vi "bd_bounds.vi"(8 "error in (no error)":errorcluster, 11 "VI Refnum":refnum<vi>) -> (0 "error out":errorcluster, 3 "VI Refnum Out":refnum<vi>)   [LabVIEW 2018]
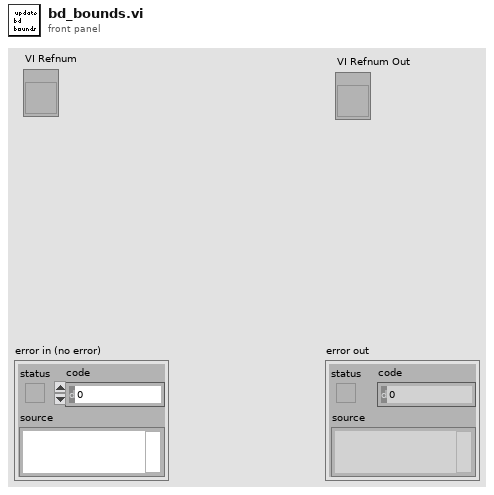
[diagram p1: front panel]
types:
  T1 = typedef "LVRectTypeDef.ctl" = cluster{"Left":i16, "Top":i16, "Right":i16, "Bottom":i16}
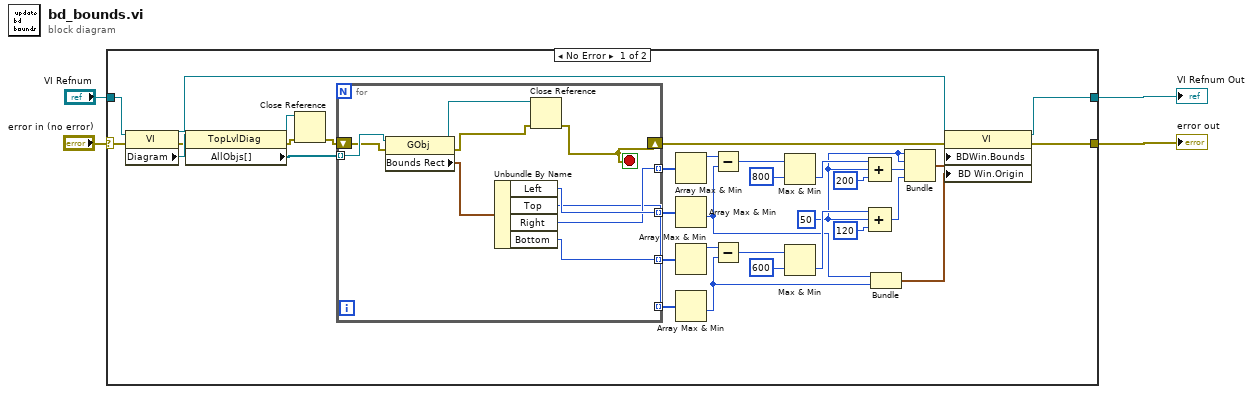
[diagram p0: block diagram]
diagram:
  n1 = case shown="No Error" "error in (no error)" {
    selector: "error in (no error)" -> [w21 w48]
    tunnel: "VI Refnum" -> [w37 w49]
    tunnel: [w12 w49] -> w3
    tunnel: [w5 w48] -> w1
    frame No Error {
      w26 = 50
      n2 = property class="VI"(reference=w37, error in=w21) -> (reference out=w29:refnum<vi>, error out=w20:errorcluster, "Diagram"=w36:refnum<vi>)
      n3 = property class="TopLvlDiag"(reference=w36, error in=w20) -> (reference out=w9:refnum<vi>, error out=w11:errorcluster, "AllObjs[]"=w35:refnum<vi>[])
      n4 = Close Reference(reference=w9, error in (no error)=w11) -> (error out=w10:errorcluster)
      n5 = for {
        tunnel: w35 -> [w47] mode=indexing
        tunnel: [w46] -> w34 mode=indexing
        tunnel: [w42] -> w33 mode=indexing
        shift-right: [w38] -> w22
        shift-left: w10 -> [w43]
        tunnel: [w45] -> w17 mode=indexing
        tunnel: [w44] -> w15 mode=indexing
        stop <- w38 stop-if-true
        n6 = property class="GObj"(reference=w47, error in=w43) -> (reference out=w39:refnum<vi>, error out=w40:errorcluster, "Bounds Rect"=w41:T1)
        n7 = Unbundle By Name(w41) -> ("Left"=w46:i16, "Top"=w42:i16, "Right"=w45:i16, "Bottom"=w44:i16)
        n8 = Close Reference(reference=w39, error in (no error)=w40) -> (error out=w38:errorcluster)
      }
      n9 = Array Max & Min(array=w17) -> (max value=w16:i16)  [unwired: 3 out]
      n10 = Array Max & Min(array=w34) -> (min value=w8:i16)  [unwired: 3 out]
      n11 = Array Max & Min(array=w15) -> (max value=w14:i16)  [unwired: 3 out]
      n12 = Array Max & Min(array=w33) -> (min value=w6:i16)  [unwired: 3 out]
      n13 = Subtract(x=w16, y=w8) -> (x-y=w32:i16)
      n14 = Subtract(x=w14, y=w6) -> (x-y=w13:i16)
      n15 = Max & Min(x=w32, y=800) -> (min(x,y)=w28:i32)  [unwired: 1 out]
      n16 = Max & Min(x=w13, y=600) -> (min(x,y)=w27:i32)  [unwired: 1 out]
      n17 = Compound Arithmetic op=ADD(w28, w26, 200 ("value")) -> (w25:i32)
      n18 = Compound Arithmetic op=ADD(w27, w26, 120 ("value")) -> (w24:i32)
      n19 = Bundle(w8, w6) -> (w7:cluster{i16, i16})  [unwired: 1 out]
      n20 = Bundle(w26, w26, w25, w24) -> (w23:cluster{i32, i32, i32, i32})  [unwired: 1 out]
      n21 = property class="VI"(reference=w29, error in=w22, "BDWin.Bounds"=w23, "BD Win.Origin"=w7) -> (reference out=w12:refnum<vi>, error out=w5:errorcluster)
    }
    frame Error {
    }
  }
  "VI Refnum Out" <- w3
  "error out" <- w1
